vi "osciloscope_config.vi"(8 "error in (no error)":errorcluster, 10 "Kalibracni bod":T1, 11 "VISA Refnum in":refnum<visa-resource-name>) -> (0 "error out":errorcluster, 3 "VISA Refnum out":refnum<visa-resource-name>)   [LabVIEW 2022 SP3]
panel:
  out "resulting string":string
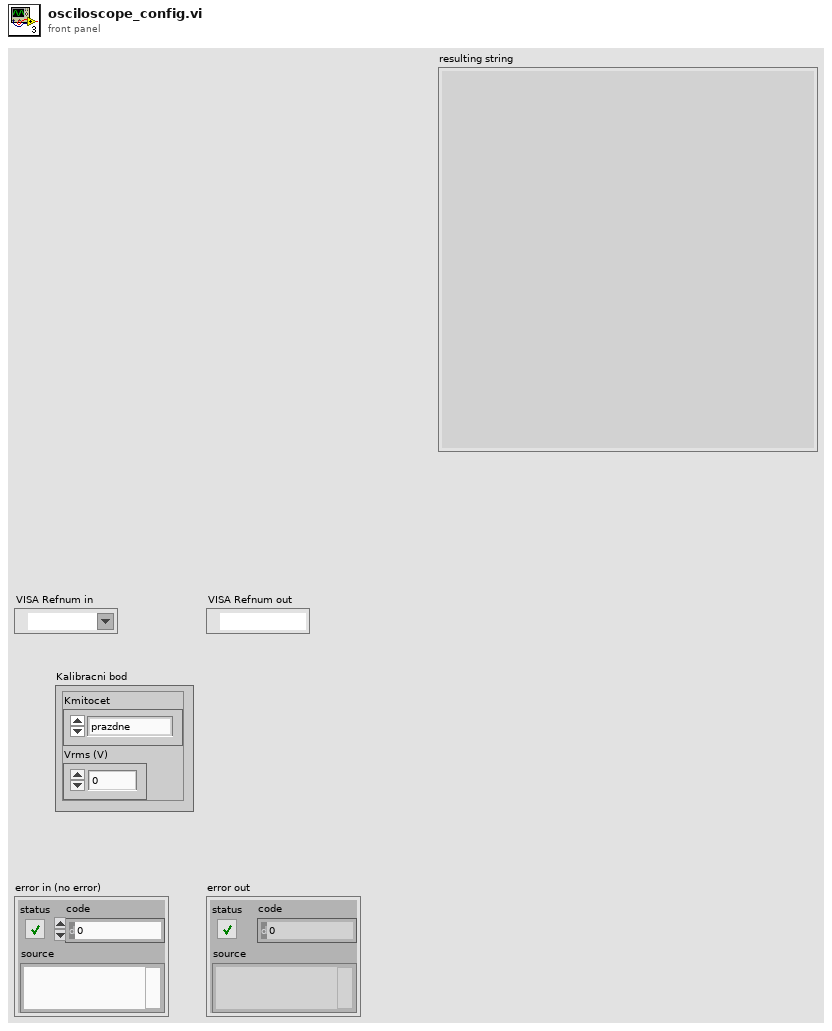
[diagram p1: front panel]
types:
  T1 = cluster{"Kmitocet":enum16{"prazdne", "50 Hz", "1 kHz", "5 kHz", "10 kHz", "20 kHz", "50 kHz", "100 kHz"}, "Vrms (V)":dbl}
  T2 = enum16{"prazdne", "50 Hz", "1 kHz", "5 kHz", "10 kHz", "20 kHz", "50 kHz", "100 kHz"}
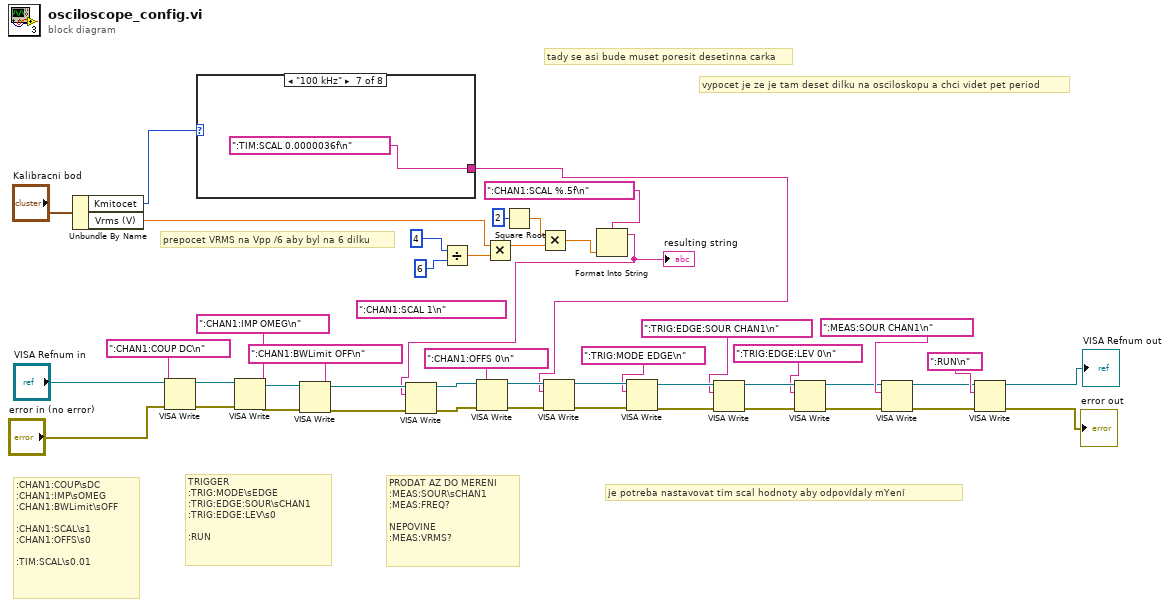
[diagram p0: block diagram]
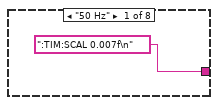
[diagram p2: hidden frame]
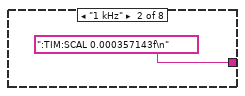
[diagram p3: hidden frame]
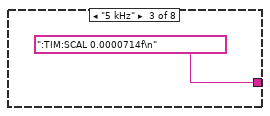
[diagram p4: hidden frame]
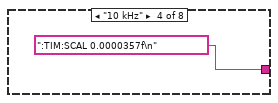
[diagram p5: hidden frame]
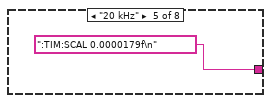
[diagram p6: hidden frame]
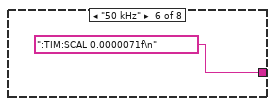
[diagram p7: hidden frame]
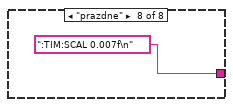
[diagram p8: hidden frame]
diagram:
  (unwired) ":CHAN1:SCAL 1\n" ("write buffer")
  # "prepocet VRMS na Vpp /6 aby byl na 6 dilku"
  # "vypocet je ze je tam deset dilku na osciloskopu a chci videt pet period"
  # "tady se asi bude muset poresit desetinna carka"
  # "je potreba nastavovat tim scal hodnoty aby odpovídaly mYení"
  # "PRODAT AZ DO MERENI\n:MEAS:SOUR\\sCHAN1\n:MEAS:FREQ?\n\nNEPOVINE\n:MEAS:VRMS?"
  # "TRIGGER\n:TRIG:MODE\\sEDGE\n:TRIG:EDGE:SOUR\\sCHAN1\n:TRIG:EDGE:LEV\\s0\n\n:RUN"
  # ":CHAN1:COUP\\sDC\n:CHAN1:IMP\\sOMEG\n:CHAN1:BWLimit\\sOFF\n\n:CHAN1:SCAL\\s1\n:CHAN1:OFFS\\s0\n\n:TIM:SCAL\\s0.01"
  n1 = Unbundle By Name("Kalibracni bod") -> ("Kmitocet"=w12:T2, "Vrms (V)"=w8:dbl)
  n2 = VISA Write(VISA resource name="VISA Refnum in", write buffer=":CHAN1:COUP DC\n", error in (no error)="error in (no error)") -> (VISA resource name out=w45:refnum<visa-resource-name>, error out=w46:errorcluster)  [unwired: 1 out]
  n3 = case shown="\"100 kHz\"" w12 {
    tunnel: [":TIM:SCAL 0.007f\n" ("format string") ":TIM:SCAL 0.000357143f\n" ("format string") ":TIM:SCAL 0.0000714f\n" ("format string") ":TIM:SCAL 0.0000357f\n" ("format string") ":TIM:SCAL 0.0000179f\n" ("format string") ":TIM:SCAL 0.0000071f\n" ("format string") ":TIM:SCAL 0.0000036f\n" ("format string") ":TIM:SCAL 0.007f\n" ("format string")] -> w1
    frame "50 Hz" {
    }
    frame "1 kHz" {
    }
    frame "5 kHz" {
    }
    frame "10 kHz" {
    }
    frame "20 kHz" {
    }
    frame "50 kHz" {
    }
    frame "100 kHz" {
    }
    frame "prazdne" {
    }
  }
  n4 = VISA Write(VISA resource name=w45, write buffer=":CHAN1:IMP OMEG\n", error in (no error)=w46) -> (VISA resource name out=w38:refnum<visa-resource-name>, error out=w37:errorcluster)  [unwired: 1 out]
  n5 = VISA Write(VISA resource name=w38, write buffer=":CHAN1:BWLimit OFF\n", error in (no error)=w37) -> (VISA resource name out=w36:refnum<visa-resource-name>, error out=w35:errorcluster)  [unwired: 1 out]
  n6 = Divide(x=4, y=6) -> (x/y=w9:dbl)
  n7 = Multiply(x=w8, y=w9) -> (x*y=w7:dbl)
  n8 = Square Root(x=2) -> (sqrt(x)=w5:dbl)
  n9 = Multiply(x=w5, y=w7) -> (x*y=w3:dbl)
  n10 = Format Into String(format string=":CHAN1:SCAL %.5f\n" ("write buffer"), w3) -> (resulting string=w2:string)  [unwired: 2 in, 1 out]
  "resulting string" <- w2
  n11 = VISA Write(VISA resource name=w36, write buffer=w2, error in (no error)=w35) -> (VISA resource name out=w34:refnum<visa-resource-name>, error out=w33:errorcluster)  [unwired: 1 out]
  n12 = VISA Write(VISA resource name=w34, write buffer=":CHAN1:OFFS 0\n", error in (no error)=w33) -> (VISA resource name out=w32:refnum<visa-resource-name>, error out=w31:errorcluster)  [unwired: 1 out]
  n13 = VISA Write(VISA resource name=w32, write buffer=w1, error in (no error)=w31) -> (VISA resource name out=w30:refnum<visa-resource-name>, error out=w29:errorcluster)  [unwired: 1 out]
  n14 = VISA Write(VISA resource name=w30, write buffer=":TRIG:MODE EDGE\n", error in (no error)=w29) -> (VISA resource name out=w27:refnum<visa-resource-name>, error out=w28:errorcluster)  [unwired: 1 out]
  n15 = VISA Write(VISA resource name=w27, write buffer=":TRIG:EDGE:SOUR CHAN1\n", error in (no error)=w28) -> (VISA resource name out=w26:refnum<visa-resource-name>, error out=w25:errorcluster)  [unwired: 1 out]
  n16 = VISA Write(VISA resource name=w26, write buffer=":TRIG:EDGE:LEV 0\n", error in (no error)=w25) -> (VISA resource name out=w17:refnum<visa-resource-name>, error out=w16:errorcluster)  [unwired: 1 out]
  n17 = VISA Write(VISA resource name=w17, write buffer=":MEAS:SOUR CHAN1\n", error in (no error)=w16) -> (VISA resource name out=w14:refnum<visa-resource-name>, error out=w15:errorcluster)  [unwired: 1 out]
  n18 = VISA Write(VISA resource name=w14, write buffer=":RUN\n", error in (no error)=w15) -> (VISA resource name out=→"VISA Refnum out":refnum<visa-resource-name>, error out=→"error out":errorcluster)  [unwired: 1 out]
